vi "step2 Solve.vi"(8 "error in (no error)":errorcluster, 11 "cube in":T1) -> (0 "error out":errorcluster, 1 "upper layer solved?":bool, 3 "cube out":T1)   [LabVIEW 2011]
doc: "Rotate cube as necessary so that the top middle piece matches the desired start colour.\n\nNo transformations are done in this VI, the operations are loaded on the the operation queue bus."
uses:
  Typedef/cube.ctl
  Typedef/face.ctl
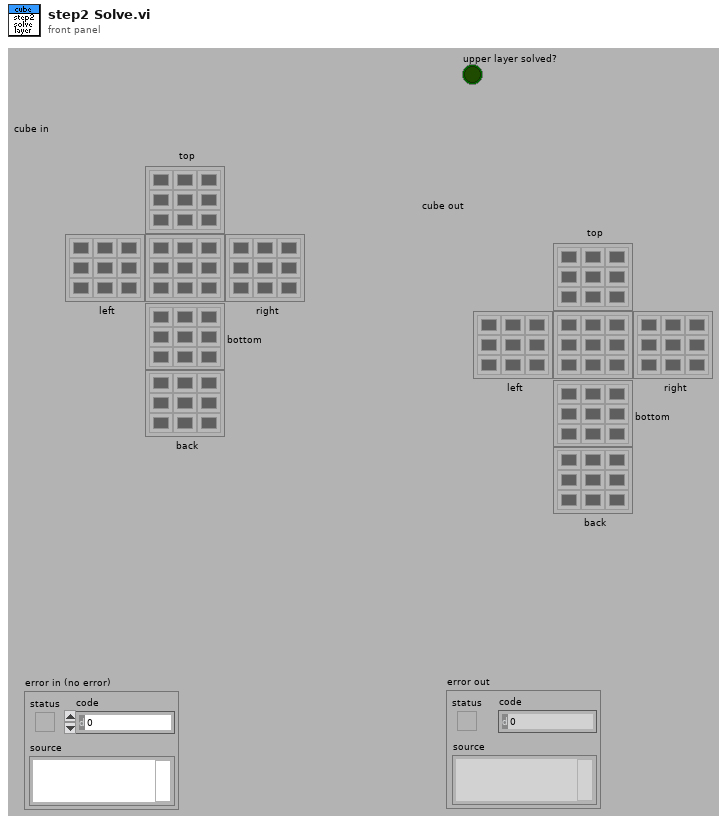
[diagram p1: front panel]
types:
  T1 = typedef "cube.ctl" = cluster{"top":T2, "left":T2, "right":T2, "bottom":T2, "back":T2, "front":T2}
  T2 = typedef "face.ctl" = u32[][]
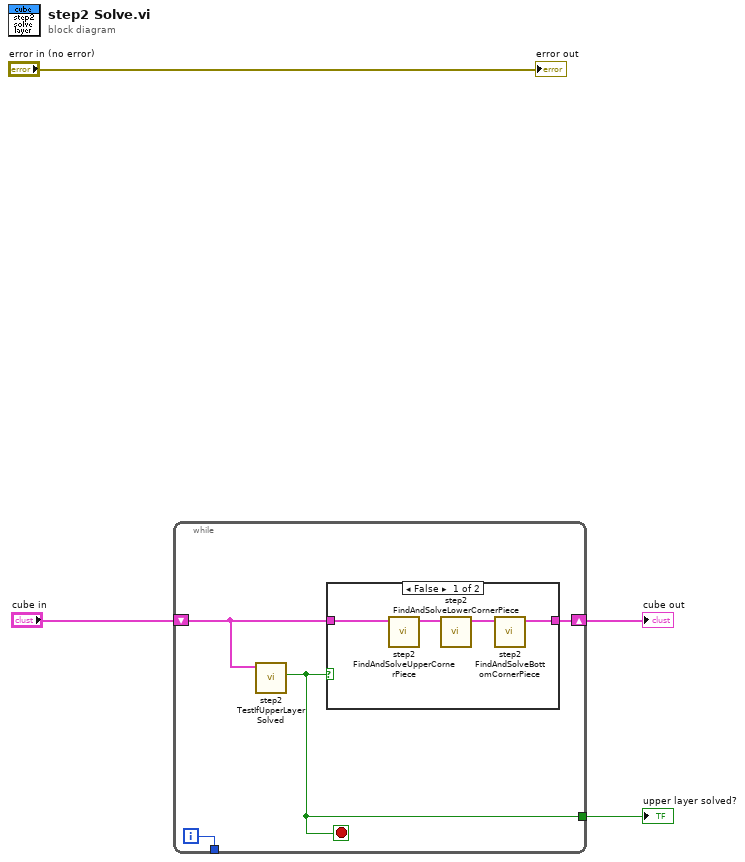
[diagram p0: block diagram]
diagram:
  n1 = while {
    shift-right: [w7] -> w2
    shift-left: "cube in" -> [w8]
    tunnel: [w6] -> w1
    tunnel: [w5] -> _
    i -> [w5]
    stop <- w6 stop-if-true
    n2 = call "step2 TestIfUpperLayerSolved.vi"("cube in"=w8) -> ("upper layer solved?"=w6:bool)  [unwired: 9 in, 1 out]
    n3 = case shown="False" w6 {
      tunnel: w8 -> [w12 w13]
      tunnel: [w9 w13] -> w7
      frame False {
        n4 = call "step2 FindAndSolveUpperCornerPiece.vi"("cube in"=w12) -> ("cube out"=w11:T1)  [unwired: 9 in, 1 out]
        n5 = call "step2 FindAndSolveLowerCornerPiece.vi"("cube in"=w11) -> ("cube out"=w10:T1)  [unwired: 9 in, 1 out]
        n6 = call "step2 FindAndSolveBottomCornerPiece.vi"("cube in"=w10) -> ("cube out"=w9:T1)  [unwired: 9 in, 1 out]
      }
      frame True {
      }
    }
  }
  "upper layer solved?" <- w1
  "cube out" <- w2
  "error out" <- "error in (no error)"
